vi "Go Home Sub_VI.vi"(8 "error in (no error)":errorcluster, 9 "stop":bool, 10 "Homing Freq":dbl format="%#_13g", 11 "Homing Duty %":dbl format="%#_13g") -> (0 "error out":errorcluster, 2 "Motor Status out":T2 {"Y Velocity (mm/s)" format="%#_3g"; "X Velocity (mm/s)" format="%#_3g"; "Homing Duty %" format="%#_13g"; "Homing Freq" format="%#_13g"})   [LabVIEW 2017]
uses:
  Go Home State type def.ctl
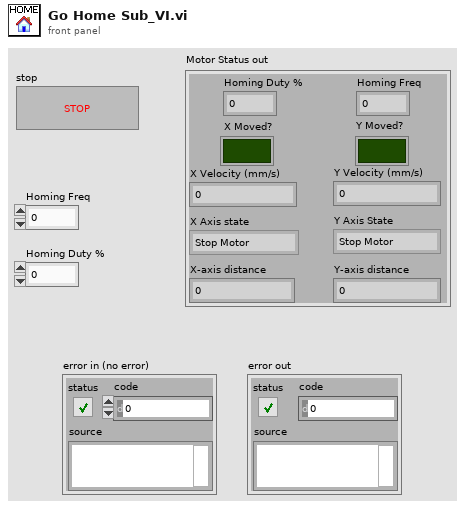
[diagram p1: front panel]
types:
  T1 = typedef "Go Home State type def.ctl" = enum16{"Stop Motor", "Read Input", "Drive Motor"}
  T2 = cluster{"Homing Freq":dbl, "Homing Duty %":dbl, "X Moved?":bool, "Y Moved?":bool, "X Axis state":T1, "Y Axis State":T1, "X-axis distance":dbl, "X Velocity (mm/s)":dbl, "Y-axis distance":dbl, "Y Velocity (mm/s)":dbl}
  T3 = typedef "Encoder Cluster.ctl" = cluster{"Y-axis rev count":dbl, "Y-axis distance":dbl, "X-axis rev count":dbl, "X-axis distance":dbl, "Y-axis direction":T4, "X-axis direction":T4, "X-counter val":i32, "Y-counter val":i32}
  T4 = typedef "Encoder Count Direction Enum.ctl" = enum16{"Counting Up", "Counting Down"}
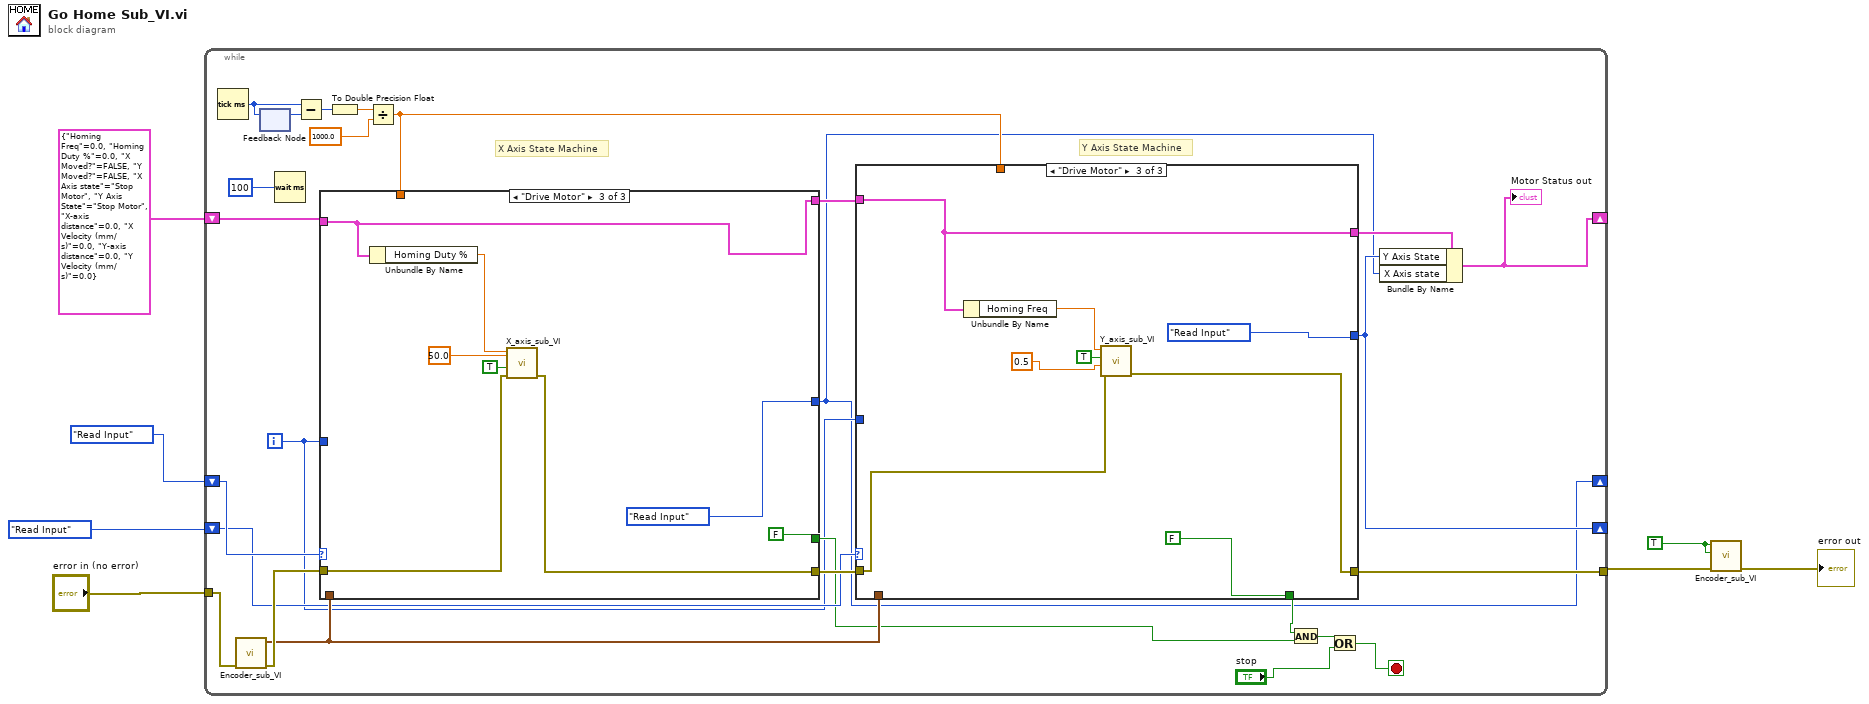
[diagram p0: block diagram]
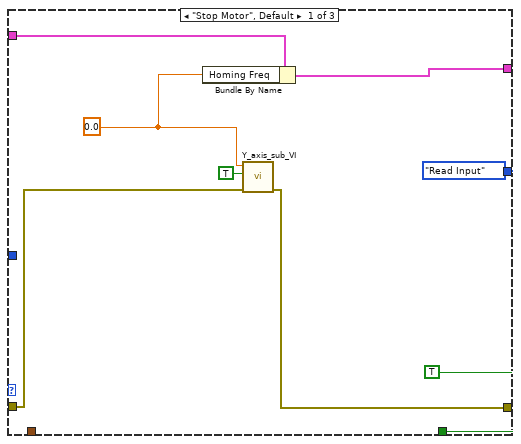
[diagram p2: hidden frame]
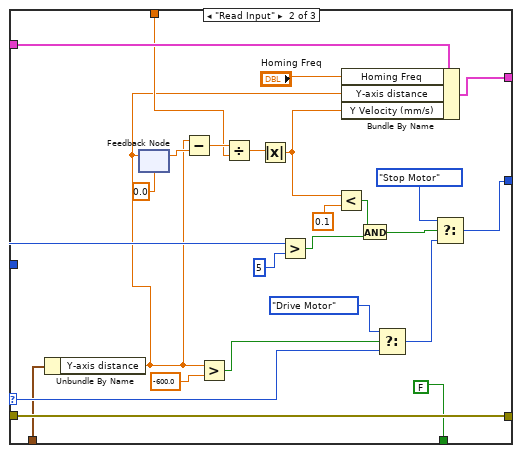
[diagram p3: hidden frame]
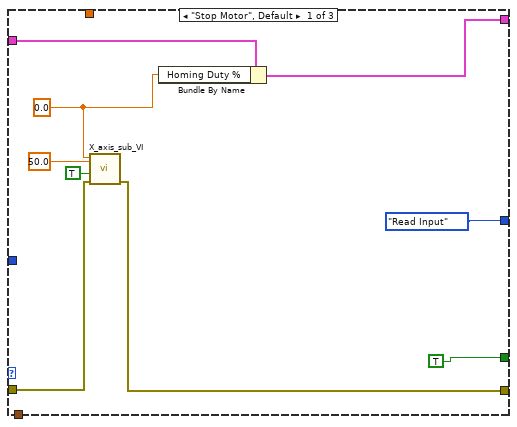
[diagram p4: hidden frame]
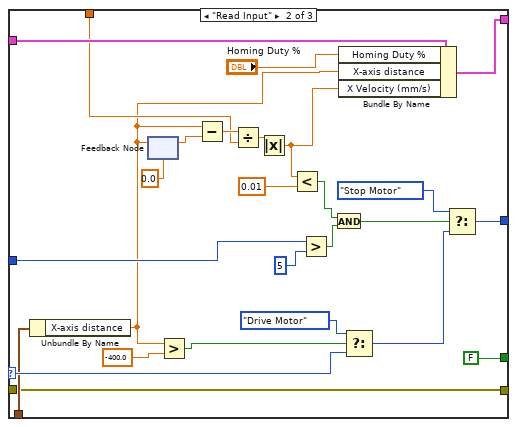
[diagram p5: hidden frame]
diagram:
  w1 = TRUE ("Reset X Counter")
  n1 = while {
    tunnel: "error in (no error)" -> [w32]
    tunnel: [w29] -> w3
    shift-right: [w8] -> _
    shift-left: Go_Home_State_type_def."Read Input" ("Enum 2") -> [w31]
    shift-right: [w10] -> _
    shift-left: T2 {"Homing Freq"=0.0, "Homing Duty %"=0.0, "X Moved?"=FALSE, "Y Moved?"=FALSE, "X Axis state"=enum."Stop Motor", "Y Axis State"=enum."Stop Motor", "X-axis distance"=0.0, "X Velocity (mm/s)"=0.0, "Y-axis distance"=0.0, "Y Velocity (mm/s)"=0.0} ("Motor Status out 2") -> [w33]
    shift-right: [w9] -> _
    shift-left: Go_Home_State_type_def."Read Input" ("Enum") -> [w25]
    i -> [w12]
    stop <- w13 stop-if-true
    # "Y Axis State Machine"
    # "X Axis State Machine"
    n2 = Tick Count (ms)() -> (millisecond timer value=w21:u32)
    n3 = call "Encoder_sub_VI.vi"("error in (no error)"=w32) -> ("error out"=w27:errorcluster, "Encoder Output"=w26:T3)  [unwired: 9 in]
    n4 = feedback-in #1(w21) -> ()
    n5 = feedback #1() -> (w20:u32)  [unwired: 1 in]
    n6 = Wait (ms)(milliseconds to wait=u32 100) -> ()  [unwired: 1 out]
    n7 = Subtract(x=w21, y=w20) -> (x-y=w19:u32)
    n8 = To Double Precision Float(number=w19) -> (double precision float=w18:dbl)
    n9 = Divide(x=w18, y=1000.0) -> (x/y=w22:dbl)
    n10 = case shown="\"Drive Motor\"" w31 {
      selector: w31 -> [_ w107 _]
      tunnel: w33 -> [w84 w102 w111]
      tunnel: [w83 w109 w111] -> w30
      tunnel: [Go_Home_State_type_def."Read Input" w103 Go_Home_State_type_def."Read Input"] -> w8
      tunnel: w27 -> [w82 w97 w116]
      tunnel: [w77 w97 w115] -> w28
      tunnel: [TRUE FALSE FALSE] -> w16
      tunnel: w26 -> [_ w105 _]
      tunnel: w22 -> [_ w88 _]
      tunnel: w12 -> [_ w96 _]
      frame "Stop Motor", Default {
        w81 = 0.0
        n11 = call "X_axis_sub_VI.vi"("error in (no error)"=w82, "FWD/RVS"=TRUE, "Frequency"=50.0, "Duty Cycle %"=w81) -> ("error out"=w77:errorcluster)  [unwired: 7 in]
        n12 = Bundle By Name(cluster=w84, "Homing Duty %"=w81) -> (w83:T2)
      }
      frame "Read Input" {
        n13 = Unbundle By Name(w105) -> ("X-axis distance"=w86:dbl)
        n14 = feedback #2(0.0 ("X-axis distance")) -> (w91:dbl)
        n15 = feedback-in #2(w86) -> ()
        n16 = Greater?(x=w86, y=-400.0) -> (0:w101:bool)
        n17 = Subtract(x=w86, y=w91) -> (x-y=w89:dbl)
        n18 = Divide(x=w89, y=w88) -> (x/y=w87:dbl)
        n19 = Absolute Value(x=w87) -> (abs(x)=w85:dbl)
        n20 = Less?(x=w85, y=0.01) -> (x < y?=w93:bool)
        n21 = Greater?(x=w96, y=5) -> (0:w94:bool)
        n22 = And(x=w93, y=w94) -> (x .and. y?=w92:bool)
        n23 = Bundle By Name(cluster=w102, "Homing Duty %"="Homing Duty %", "X-axis distance"=w86, "X Velocity (mm/s)"=w85) -> (w109:T2)
        n24 = Select(t=Go_Home_State_type_def."Drive Motor", s=w101, f=w107) -> (s? t:f=w100:T1)
        n25 = Select(t=Go_Home_State_type_def."Stop Motor", s=w92, f=w100) -> (s? t:f=w103:T1)
      }
      frame "Drive Motor" {
        n26 = Unbundle By Name(w111) -> ("Homing Duty %"=w114:dbl)
        n27 = call "X_axis_sub_VI.vi"("error in (no error)"=w116, "FWD/RVS"=TRUE, "Frequency"=50.0, "Duty Cycle %"=w114) -> ("error out"=w115:errorcluster)  [unwired: 7 in]
      }
    }
    n28 = case shown="\"Drive Motor\"" w25 {
      selector: w25 -> [_ w65 _]
      tunnel: [w41 w67 w69] -> w11
      tunnel: [Go_Home_State_type_def."Read Input" w63 Go_Home_State_type_def."Read Input"] -> w9
      tunnel: w28 -> [w34 w60 w73]
      tunnel: [w40 w60 w72] -> w29
      tunnel: [TRUE FALSE FALSE ("stop")] -> w17
      tunnel: w30 -> [w35 w58 w69]
      tunnel: w26 -> [_ w59 _]
      tunnel: w22 -> [_ w48 _]
      tunnel: w12 -> [_ w44 _]
      frame "Stop Motor", Default {
        w39 = 0.0
        n29 = Bundle By Name(cluster=w35, "Homing Freq"=w39) -> (w41:T2)
        n30 = call "Y_axis_sub_VI.vi"("error in (no error)"=w34, "FWD/RVS"=TRUE, "Frequency"=w39) -> ("error out"=w40:errorcluster)  [unwired: 8 in]
      }
      frame "Read Input" {
        n31 = Unbundle By Name(w59) -> ("Y-axis distance"=w42:dbl)
        n32 = feedback #3(0.0 ("X-axis distance")) -> (w49:dbl)
        n33 = feedback-in #3(w42) -> ()
        n34 = Subtract(x=w42, y=w49) -> (x-y=w50:dbl)
        n35 = Greater?(x=w42, y=-600.0) -> (0:w56:bool)
        n36 = Divide(x=w50, y=w48) -> (x/y=w51:dbl)
        n37 = Absolute Value(x=w51) -> (abs(x)=w43:dbl)
        n38 = Greater?(x=w44, y=5) -> (0:w45:bool)
        n39 = Less?(x=w43, y=0.1) -> (x < y?=w53:bool)
        n40 = Bundle By Name(cluster=w58, "Homing Freq"="Homing Freq", "Y-axis distance"=w42, "Y Velocity (mm/s)"=w43) -> (w67:T2)
        n41 = And(x=w53, y=w45) -> (x .and. y?=w54:bool)
        n42 = Select(t=Go_Home_State_type_def."Drive Motor", s=w56, f=w65) -> (s? t:f=w57:T1)
        n43 = Select(t=Go_Home_State_type_def."Stop Motor", s=w54, f=w57) -> (s? t:f=w63:T1)
      }
      frame "Drive Motor" {
        n44 = Unbundle By Name(w69) -> ("Homing Freq"=w70:dbl)
        n45 = call "Y_axis_sub_VI.vi"("error in (no error)"=w73, "Duty Cycle"=0.5, "FWD/RVS"=TRUE, "Frequency"=w70) -> ("error out"=w72:errorcluster)  [unwired: 7 in]
      }
    }
    n46 = And(x=w17, y=w16) -> (x .and. y?=w15:bool)
    n47 = Or(x=w15, y="stop") -> (x .or. y?=w13:bool)
    n48 = Bundle By Name(cluster=w11, "Y Axis State"=w9, "X Axis state"=w8) -> (w10:T2)
    "Motor Status out" <- w10
  }
  n49 = call "Encoder_sub_VI.vi"("error in (no error)"=w3, "Reset Y Counter"=w1, "Reset X Counter"=w1) -> ("error out"=→"error out":errorcluster)  [unwired: 7 in, 1 out]
